vi "Control.vi"() -> ()   [LabVIEW 2020]
uses:
  proceso1.vi
  proceso2.vi
  proceso3.vi
  proceso4.vi
  proceso5.vi
  proceso6.vi
panel:
  in  "Numeric 14":dbl
  in  "Numeric 13":dbl
  in  "Numeric 12":dbl
  in  "Numeric 11":dbl
  in  "Numeric 10":dbl
  out "Boolean":bool
  in  "Numeric 9":dbl
  in  "Numeric 8":dbl
  in  "Numeric 7":dbl
  in  "Numeric 6":dbl
  in  "Numeric 5":dbl
  in  "Numeric 4":dbl
  in  "Numeric 3":dbl
  in  "Numeric 2":dbl
  out "s? t:f":dbl
  in  "Numeric":dbl
types:
  T1 = typedef "Semaphore RefNum" = refnum<k1>
  T2 = cluster{"final_linea":bool, "vent 1":bool, "vent 2":bool, "vent 3":bool, "mov caja 2 horizontal":i32, "llenado caja 2":u8, "pos_inicial_horizontal":dbl, " pos_final_horizontal":dbl, "contador":dbl, "mov caja 2  vertical":i32, "pos_inicial_vertical":dbl, " pos_final_vertical":dbl}
  T3 = cluster{"sensor_refrigerador":bool, "temperatura":dbl, "tuberia 5":u8, "tuberia 6":u8}
  T4 = cluster{"sensor_intercambiador":bool, "sensor_caldera":bool, "sensor_bomba_2 ":bool, "tuberia 2":u8, "tuberia 3":u8, "tuberia 4":u8, "temperatura":dbl}
  T5 = cluster{"sensor_bomba_1":bool, "tanque in":u8, " tuberia 1":u8}
  T6 = cluster{"sensor_caja":bool, "vent 1":bool, "vent 2":bool, "vent 3":bool, "pos_inicial":dbl, "pos_final":dbl, "mov_caja 1":i32}
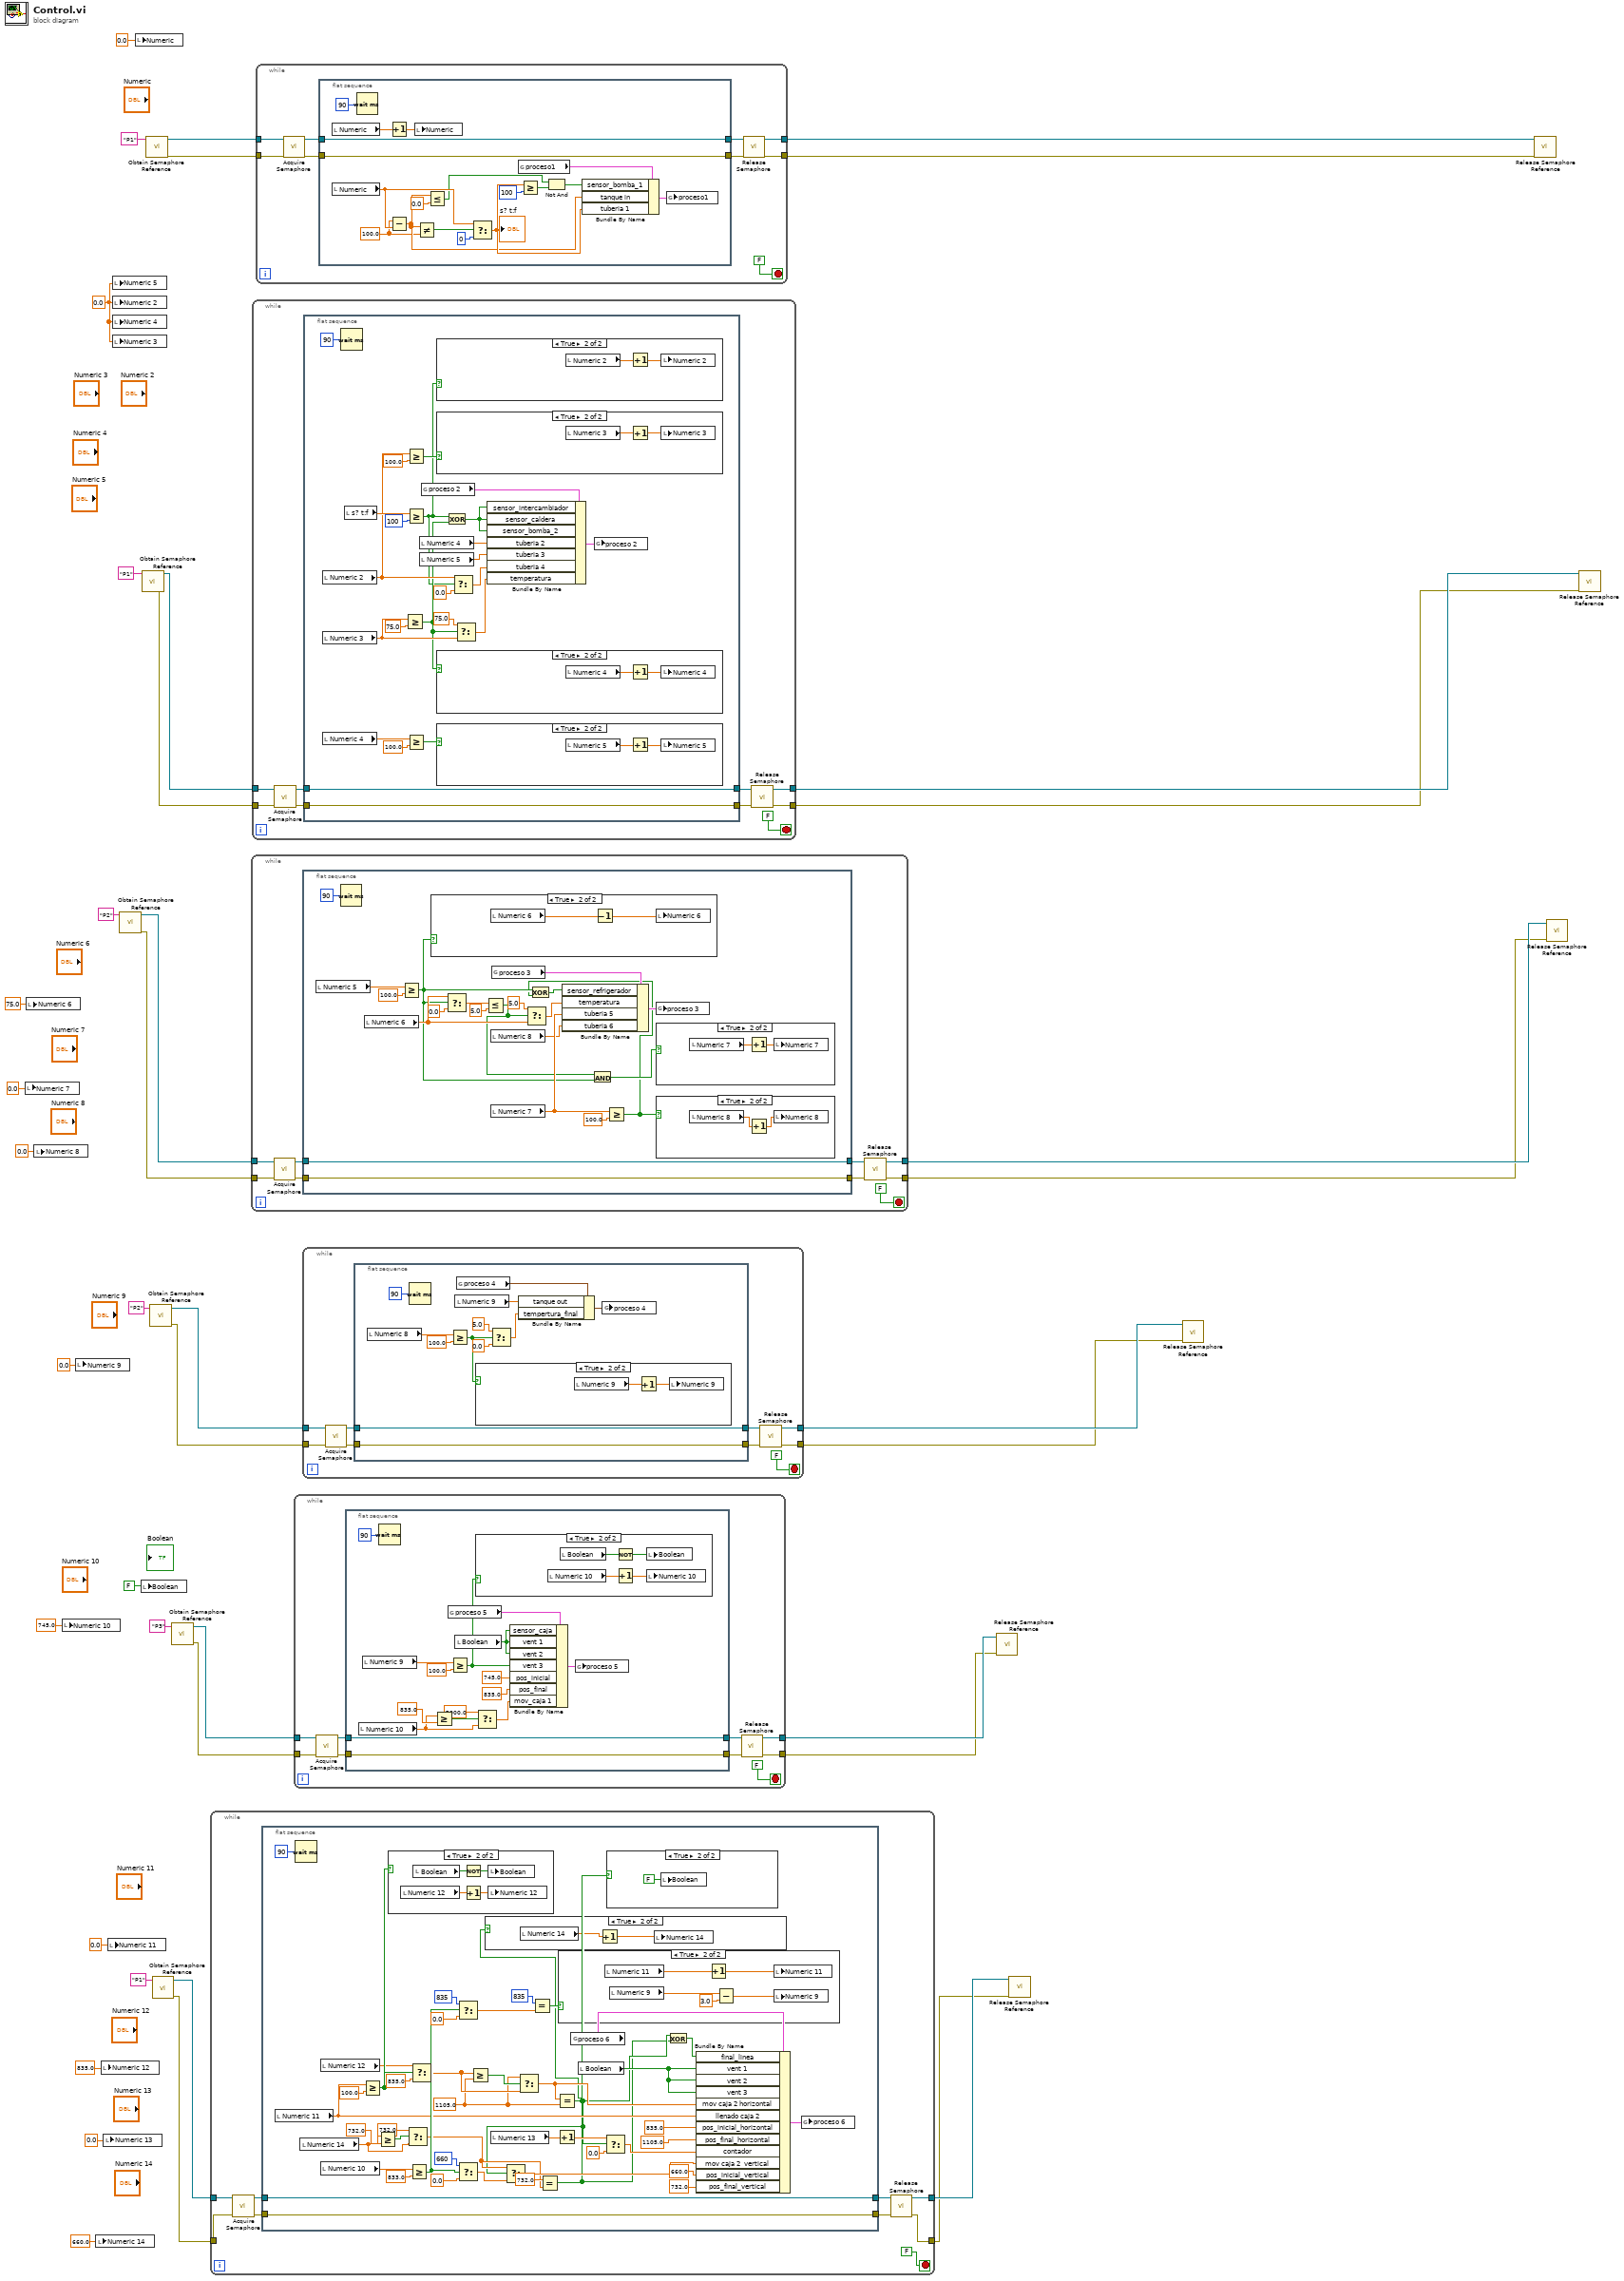
[diagram p0: block diagram]
diagram:
  w31 = 0.0 ("Numeric 2")
  n1 = local write "Numeric 7"(0.0 ("Numeric 7")) -> ()
  n2 = local write "Numeric 6"(75.0 ("Numeric 6")) -> ()
  n3 = local write "Numeric 8"(0.0 ("Numeric 8")) -> ()
  n4 = local write "Numeric 10"(745.0 ("Numeric 10")) -> ()
  n5 = local write "Numeric 9"(0.0 ("Numeric 9")) -> ()
  n6 = local write "Numeric 14"(660.0 ("Numeric 14")) -> ()
  n7 = local write "Numeric 12"(835.0 ("Numeric 12")) -> ()
  n8 = local write "Numeric 13"(0.0 ("Numeric 13")) -> ()
  n9 = local write "Numeric 11"(0.0 ("Numeric 11")) -> ()
  n10 = local write "Numeric 5"(w31) -> ()
  n11 = local write "Numeric 2"(w31) -> ()
  n12 = local write "Numeric 4"(w31) -> ()
  n13 = local write "Numeric 3"(w31) -> ()
  n14 = call <vilib>:"Obtain Semaphore Reference.vi"("name (unnamed)"="P2") -> ("error out"=w29:errorcluster, "semaphore"=w30:T1)  [unwired: 4 in, 1 out]
  n15 = local write "Numeric"(0.0 ("Numeric")) -> ()
  n16 = local write "Boolean"(FALSE ("Boolean")) -> ()
  n17 = call <vilib>:"Obtain Semaphore Reference.vi"("name (unnamed)"="P1") -> ("error out"=w33:errorcluster, "semaphore"=w32:T1)  [unwired: 4 in, 1 out]
  n18 = call <vilib>:"Obtain Semaphore Reference.vi"("name (unnamed)"="P1") -> ("error out"=w35:errorcluster, "semaphore"=w34:T1)  [unwired: 4 in, 1 out]
  n19 = call <vilib>:"Obtain Semaphore Reference.vi"("name (unnamed)"="P2") -> ("error out"=w21:errorcluster, "semaphore"=w22:T1)  [unwired: 4 in, 1 out]
  n20 = call <vilib>:"Obtain Semaphore Reference.vi"("name (unnamed)"="P1") -> ("error out"=w9:errorcluster, "semaphore"=w10:T1)  [unwired: 4 in, 1 out]
  n21 = call <vilib>:"Obtain Semaphore Reference.vi"("name (unnamed)"="P3") -> ("error out"=w16:errorcluster, "semaphore"=w17:T1)  [unwired: 4 in, 1 out]
  n22 = while {
    tunnel: w10 -> [w50]
    tunnel: w9 -> [w49]
    tunnel: [w44] -> w8
    tunnel: [w43] -> w7
    stop <- FALSE stop-if-true
    n23 = call <vilib>:"Acquire Semaphore.vi"("error in (no error)"=w49, "semaphore"=w50) -> ("error out"=w46:errorcluster, "semaphore out"=w48:T1)  [unwired: 3 in, 1 out]
    n24 = flat-sequence {
      tunnel: w48 -> [w84]
      tunnel: [w84] -> w47
      tunnel: w46 -> [w92]
      tunnel: [w92] -> w45
      frame #0 {
        w67 = 1105.0 ("y")
        n25 = local read "Numeric 11"() -> (w76:dbl)
        n26 = Wait (ms)(milliseconds to wait=u32 90) -> ()  [unwired: 1 out]
        n27 = local read "Numeric 14"() -> (w59:dbl)
        n28 = local read "Numeric 12"() -> (w71:dbl)
        n29 = local read "Numeric 10"() -> (w89:dbl)
        n30 = Greater Or Equal?(x=w76, y=100.0) -> (x >= y?=w72:bool)
        n31 = Greater Or Equal?(x=w59, y=732.0) -> (x >= y?=w61:bool)
        n32 = case shown="True" w72 {
          frame False {
          }
          frame True {
            n33 = local read "Numeric 12"() -> (w102:dbl)
            n34 = local read "Boolean"() -> (w99:bool)
            n35 = Not(x=w99) -> (.not. x?=w100:bool)
            n36 = Increment(x=w102) -> (x+1=w101:dbl)
            n37 = local write "Boolean"(w100) -> ()
            n38 = local write "Numeric 12"(w101) -> ()
          }
        }
        n39 = Select(t=732.0, s=w61, f=w59) -> (s? t:f=w55:dbl)
        n40 = Greater Or Equal?(x=w89, y=833.0) -> (x >= y?=w86:bool)
        n41 = Select(t=w71, s=w72, f=835.0) -> (s? t:f=w69:dbl)
        n42 = Select(t=835 ("mov caja 2 horizontal"), s=w86, f=0.0) -> (s? t:f=w74:dbl)
        n43 = Select(t=660 ("mov caja 2  vertical"), s=w86, f=0.0) -> (s? t:f=w58:dbl)
        n44 = Greater Or Equal?(x=w69, y=w67) -> (x >= y?=w70:bool)
        n45 = local read "Numeric 13"() -> (w66:dbl)
        n46 = Select(t=w67, s=w70, f=w69) -> (s? t:f=w68:dbl)
        n47 = Equal?(x=835, y=w74) -> (x = y?=w78:bool)
        n48 = Equal?(x=732.0, y=w55) -> (x = y?=w53:bool)
        n49 = Equal?(x=w68, y=w67) -> (x = y?=w54:bool)
        n50 = case shown="True" w54 {
          frame False {
          }
          frame True {
            n51 = local read "Numeric 14"() -> (w97:dbl)
            n52 = Increment(x=w97) -> (x+1=w98:dbl)
            n53 = local write "Numeric 14"(w98) -> ()
          }
        }
        n54 = Select(t=w55, s=w54, f=w58) -> (s? t:f=w57:dbl)
        n55 = Increment(x=w66) -> (x+1=w65:dbl)
        n56 = case shown="True" w78 {
          frame False {
          }
          frame True {
            n57 = local read "Numeric 11"() -> (w107:dbl)
            n58 = local read "Numeric 9"() -> (w105:dbl)
            n59 = Increment(x=w107) -> (x+1=w106:dbl)
            n60 = Subtract(x=w105, y=3.0) -> (x-y=w104:dbl)
            n61 = local write "Numeric 11"(w106) -> ()
            n62 = local write "Numeric 9"(w104) -> ()
          }
        }
        n63 = global read "proceso6.vi" "proceso 6"() -> (w95:T2)
        n64 = local read "Boolean"() -> (w93:bool)
        n65 = Select(t=w65, s=w54, f=0.0) -> (s? t:f=w63:dbl)
        n66 = case shown="True" w53 {
          frame False {
          }
          frame True {
            n67 = local write "Boolean"(FALSE ("Boolean")) -> ()
          }
        }
        n68 = Exclusive Or(1:w53, 2:w54) -> (0:w52:bool)
        n69 = Bundle By Name(cluster=w95, "final_linea"=w52, "vent 1"=w93, "vent 2"=w93, "vent 3"=w93, "mov caja 2 horizontal"=w68, "llenado caja 2"=w76, "pos_inicial_horizontal"=835.0, "pos_final_horizontal"=1105.0, "contador"=w63, "mov caja 2  vertical"=w57, "pos_inicial_vertical"=660.0, "pos_final_vertical"=732.0) -> (w94:T2)
        n70 = global write "proceso6.vi" "proceso 6"(w94) -> ()
      }
    }
    n71 = call <vilib>:"Release Semaphore.vi"("error in (no error)"=w45, "semaphore"=w47) -> ("error out"=w43:errorcluster, "semaphore out"=w44:T1)  [unwired: 4 in]
  }
  n72 = while {
    tunnel: w30 -> [w115]
    tunnel: w29 -> [w114]
    tunnel: [w109] -> w28
    tunnel: [w108] -> w27
    stop <- FALSE stop-if-true
    n73 = call <vilib>:"Acquire Semaphore.vi"("error in (no error)"=w114, "semaphore"=w115) -> ("error out"=w112:errorcluster, "semaphore out"=w113:T1)  [unwired: 3 in, 1 out]
    n74 = flat-sequence {
      tunnel: w113 -> [w133]
      tunnel: w112 -> [w132]
      tunnel: [w133] -> w111
      tunnel: [w132] -> w110
      frame #0 {
        n75 = local read "Numeric 5"() -> (w135:dbl)
        n76 = Wait (ms)(milliseconds to wait=u32 90) -> ()  [unwired: 1 out]
        n77 = local read "Numeric 6"() -> (w126:dbl)
        n78 = Greater Or Equal?(x=w135, y=100.0) -> (x >= y?=w119:bool)
        n79 = case shown="True" w119 {
          frame False {
          }
          frame True {
            n80 = local read "Numeric 6"() -> (w143:dbl)
            n81 = Decrement(x=w143) -> (x-1=w142:dbl)
            n82 = local write "Numeric 6"(w142) -> ()
          }
        }
        n83 = Select(t=w126, s=w119, f=0.0) -> (s? t:f=w129:dbl)
        n84 = Less Or Equal?(x=w129, y=5.0) -> (x <= y?=w121:bool)
        n85 = local read "Numeric 8"() -> (w123:dbl)
        n86 = local read "Numeric 7"() -> (w124:dbl)
        n87 = global read "proceso3.vi" "proceso 3"() -> (w137:T3)
        n88 = Select(t=5.0, s=w121, f=w126) -> (s? t:f=w122:dbl)
        n89 = And(x=w121, y=w119) -> (x .and. y?=w120:bool)
        n90 = Greater Or Equal?(x=w124, y=100.0) -> (x >= y?=w118:bool)
        n91 = Exclusive Or(1:w118, 2:w119) -> (0:w117:bool)
        n92 = Bundle By Name(cluster=w137, "sensor_refrigerador"=w117, "temperatura"=w122, "tuberia 5"=w124, "tuberia 6"=w123) -> (w136:T3)
        n93 = global write "proceso3.vi" "proceso 3"(w136) -> ()
        n94 = case shown="True" w120 {
          frame False {
          }
          frame True {
            n95 = local read "Numeric 7"() -> (w141:dbl)
            n96 = Increment(x=w141) -> (x+1=w140:dbl)
            n97 = local write "Numeric 7"(w140) -> ()
          }
        }
        n98 = case shown="True" w118 {
          frame False {
          }
          frame True {
            n99 = local read "Numeric 8"() -> (w139:dbl)
            n100 = Increment(x=w139) -> (x+1=w138:dbl)
            n101 = local write "Numeric 8"(w138) -> ()
          }
        }
      }
    }
    n102 = call <vilib>:"Release Semaphore.vi"("error in (no error)"=w110, "semaphore"=w111) -> ("error out"=w108:errorcluster, "semaphore out"=w109:T1)  [unwired: 4 in]
  }
  n103 = while {
    tunnel: [w151] -> w40
    tunnel: [w150] -> w39
    tunnel: w33 -> [w149]
    tunnel: w32 -> [w148]
    stop <- FALSE stop-if-true
    n104 = call <vilib>:"Acquire Semaphore.vi"("error in (no error)"=w149, "semaphore"=w148) -> ("error out"=w146:errorcluster, "semaphore out"=w147:T1)  [unwired: 3 in, 1 out]
    n105 = flat-sequence {
      tunnel: w147 -> [w170]
      tunnel: w146 -> [w169]
      tunnel: [w170] -> w145
      tunnel: [w169] -> w144
      frame #0 {
        n106 = local read "Numeric 2"() -> (w163:dbl)
        n107 = local read "Numeric 3"() -> (w164:dbl)
        n108 = local read "Numeric 4"() -> (w159:dbl)
        n109 = Wait (ms)(milliseconds to wait=u32 90) -> ()  [unwired: 1 out]
        n110 = local read "s? t:f"() -> (w174:dbl)
        n111 = Greater Or Equal?(x=w164, y=75.0) -> (x >= y?=w155:bool)
        n112 = Greater Or Equal?(x=w163, y=100.0 ("x")) -> (x >= y?=w161:bool)
        n113 = Greater Or Equal?(x=w174, y=100) -> (x >= y?=w154:bool)
        n114 = Greater Or Equal?(x=w159, y=100.0) -> (x >= y?=w160:bool)
        n115 = local read "Numeric 4"() -> (w157:dbl)
        n116 = local read "Numeric 5"() -> (w156:dbl)
        n117 = global read "proceso2.vi" "proceso 2"() -> (w175:T4)
        n118 = case shown="True" w154 {
          frame False {
          }
          frame True {
            n119 = local read "Numeric 2"() -> (w183:dbl)
            n120 = Increment(x=w183) -> (x+1=w184:dbl)
            n121 = local write "Numeric 2"(w184) -> ()
          }
        }
        n122 = case shown="True" w161 {
          frame False {
          }
          frame True {
            n123 = local read "Numeric 3"() -> (w181:dbl)
            n124 = Increment(x=w181) -> (x+1=w182:dbl)
            n125 = local write "Numeric 3"(w182) -> ()
          }
        }
        n126 = case shown="True" w155 {
          frame False {
          }
          frame True {
            n127 = local read "Numeric 4"() -> (w180:dbl)
            n128 = Increment(x=w180) -> (x+1=w179:dbl)
            n129 = local write "Numeric 4"(w179) -> ()
          }
        }
        n130 = case shown="True" w160 {
          frame False {
          }
          frame True {
            n131 = local read "Numeric 5"() -> (w178:dbl)
            n132 = Increment(x=w178) -> (x+1=w177:dbl)
            n133 = local write "Numeric 5"(w177) -> ()
          }
        }
        n134 = Exclusive Or(1:w155, 2:w154) -> (0:w153:bool)
        n135 = Select(t=w163, s=w154, f=0.0) -> (s? t:f=w171:dbl)
        n136 = Select(t=75.0, s=w155, f=w164) -> (s? t:f=w166:dbl)
        n137 = Bundle By Name(cluster=w175, "sensor_intercambiador"=w153, "sensor_caldera"=w153, "sensor_bomba_2"=w153, "tuberia 2"=w157, "tuberia 3"=w156, "tuberia 4"=w171, "temperatura"=w166) -> (w176:T4)
        n138 = global write "proceso2.vi" "proceso 2"(w176) -> ()
      }
    }
    n139 = call <vilib>:"Release Semaphore.vi"("error in (no error)"=w144, "semaphore"=w145) -> ("error out"=w150:errorcluster, "semaphore out"=w151:T1)  [unwired: 4 in]
  }
  n140 = while {
    tunnel: [w192] -> w37
    tunnel: [w191] -> w36
    tunnel: w35 -> [w188]
    tunnel: w34 -> [w187]
    stop <- FALSE stop-if-true
    n141 = call <vilib>:"Acquire Semaphore.vi"("error in (no error)"=w188, "semaphore"=w187) -> ("error out"=w186:errorcluster, "semaphore out"=w185:T1)  [unwired: 3 in, 1 out]
    n142 = flat-sequence {
      tunnel: w185 -> [w195]
      tunnel: [w195] -> w190
      tunnel: w186 -> [w194]
      tunnel: [w194] -> w189
      frame #0 {
        w196 = 100.0 ("x")
        n143 = local read "Numeric"() -> (w209:dbl)
        n144 = local read "Numeric"() -> (w211:dbl)
        n145 = Wait (ms)(milliseconds to wait=u32 90) -> ()  [unwired: 1 out]
        n146 = Increment(x=w209) -> (x+1=w210:dbl)
        n147 = Subtract(x=w196, y=w211) -> (x-y=w204:dbl)
        n148 = local write "Numeric"(w210) -> ()
        n149 = Not Equal?(x=w204, y=w196) -> (x != y?=w203:bool)
        n150 = Less Or Equal?(x=w204, y=0.0) -> (x <= y?=w205:bool)
        n151 = Select(t=w211, s=w203, f=0) -> (s? t:f=w208:dbl)
        "s? t:f" <- w208
        n152 = global read "proceso1.vi" "proceso1"() -> (w201:T5)
        n153 = Greater Or Equal?(x=w208, y=100) -> (x >= y?=w206:bool)
        n154 = Not And(1:w206, 2:w205) -> (0:w207:bool)
        n155 = Bundle By Name(cluster=w201, "sensor_bomba_1"=w207, "tanque in"=w204, "tuberia 1"=w208) -> (w202:T5)
        n156 = global write "proceso1.vi" "proceso1"(w202) -> ()
      }
    }
    n157 = call <vilib>:"Release Semaphore.vi"("error in (no error)"=w189, "semaphore"=w190) -> ("error out"=w192:errorcluster, "semaphore out"=w191:T1)  [unwired: 4 in]
  }
  n158 = while {
    tunnel: w17 -> [w219]
    tunnel: w16 -> [w218]
    tunnel: [w213] -> w15
    tunnel: [w212] -> w14
    stop <- FALSE stop-if-true
    n159 = call <vilib>:"Acquire Semaphore.vi"("error in (no error)"=w218, "semaphore"=w219) -> ("error out"=w216:errorcluster, "semaphore out"=w217:T1)  [unwired: 3 in, 1 out]
    n160 = flat-sequence {
      tunnel: w217 -> [w232]
      tunnel: w216 -> [w231]
      tunnel: [w232] -> w215
      tunnel: [w231] -> w214
      frame #0 {
        n161 = local read "Numeric 10"() -> (w223:dbl)
        n162 = local read "Numeric 9"() -> (w233:dbl)
        n163 = Wait (ms)(milliseconds to wait=u32 90) -> ()  [unwired: 1 out]
        n164 = Greater Or Equal?(x=w223, y=835.0) -> (x >= y?=w225:bool)
        n165 = global read "proceso5.vi" "proceso 5"() -> (w236:T6)
        n166 = Greater Or Equal?(x=w233, y=100.0) -> (x >= y?=w229:bool)
        n167 = local read "Boolean"() -> (w228:bool)
        n168 = case shown="True" w229 {
          frame False {
          }
          frame True {
            n169 = local read "Numeric 10"() -> (w237:dbl)
            n170 = local read "Boolean"() -> (w239:bool)
            n171 = Not(x=w239) -> (.not. x?=w240:bool)
            n172 = Increment(x=w237) -> (x+1=w238:dbl)
            n173 = local write "Boolean"(w240) -> ()
            n174 = local write "Numeric 10"(w238) -> ()
          }
        }
        n175 = Select(t=2000.0, s=w225, f=w223) -> (s? t:f=w222:dbl)
        n176 = Bundle By Name(cluster=w236, "sensor_caja"=w228, "vent 1"=w228, "vent 2"=w228, "vent 3"=w229, "pos_inicial"=745.0, "pos_final"=835.0, "mov_caja 1"=w222) -> (w235:T6)
        n177 = global write "proceso5.vi" "proceso 5"(w235) -> ()
      }
    }
    n178 = call <vilib>:"Release Semaphore.vi"("error in (no error)"=w214, "semaphore"=w215) -> ("error out"=w212:errorcluster, "semaphore out"=w213:T1)  [unwired: 4 in]
  }
  n179 = while {
    tunnel: w22 -> [w248]
    tunnel: w21 -> [w247]
    tunnel: [w242] -> w20
    tunnel: [w241] -> w19
    stop <- FALSE stop-if-true
    n180 = call <vilib>:"Acquire Semaphore.vi"("error in (no error)"=w247, "semaphore"=w248) -> ("error out"=w245:errorcluster, "semaphore out"=w246:T1)  [unwired: 3 in, 1 out]
    n181 = flat-sequence {
      tunnel: w246 -> [w259]
      tunnel: w245 -> [w258]
      tunnel: [w259] -> w244
      tunnel: [w258] -> w243
      frame #0 {
        n182 = local read "Numeric 8"() -> (w257:dbl)
        n183 = Wait (ms)(milliseconds to wait=u32 90) -> ()  [unwired: 1 out]
        n184 = Greater Or Equal?(x=w257, y=100.0) -> (x >= y?=w254:bool)
        n185 = local read "Numeric 9"() -> (w255:dbl)
        n186 = global read "proceso4.vi" "proceso 4"() -> (w261:cluster{"tanque out":u8, "tempertura_final":dbl})
        n187 = case shown="True" w254 {
          frame False {
          }
          frame True {
            n188 = local read "Numeric 9"() -> (w263:dbl)
            n189 = Increment(x=w263) -> (x+1=w262:dbl)
            n190 = local write "Numeric 9"(w262) -> ()
          }
        }
        n191 = Select(t=5.0, s=w254, f=0.0) -> (s? t:f=w253:dbl)
        n192 = Bundle By Name(cluster=w261, "tanque out"=w255, "tempertura_final"=w253) -> (w260:cluster{"tanque out":u8, "tempertura_final":dbl})
        n193 = global write "proceso4.vi" "proceso 4"(w260) -> ()
      }
    }
    n194 = call <vilib>:"Release Semaphore.vi"("error in (no error)"=w243, "semaphore"=w244) -> ("error out"=w241:errorcluster, "semaphore out"=w242:T1)  [unwired: 4 in]
  }
  n195 = call <vilib>:"Release Semaphore Reference.vi"("error in (no error)"=w14, "semaphore"=w15) -> ()  [unwired: 8 in, 2 out]
  n196 = call <vilib>:"Release Semaphore Reference.vi"("error in (no error)"=w7, "semaphore"=w8) -> ()  [unwired: 8 in, 2 out]
  n197 = call <vilib>:"Release Semaphore Reference.vi"("error in (no error)"=w19, "semaphore"=w20) -> ()  [unwired: 8 in, 2 out]
  n198 = call <vilib>:"Release Semaphore Reference.vi"("error in (no error)"=w37, "semaphore"=w36) -> ()  [unwired: 8 in, 2 out]
  n199 = call <vilib>:"Release Semaphore Reference.vi"("error in (no error)"=w27, "semaphore"=w28) -> ()  [unwired: 8 in, 2 out]
  n200 = call <vilib>:"Release Semaphore Reference.vi"("error in (no error)"=w39, "semaphore"=w40) -> ()  [unwired: 8 in, 2 out]
